vi "Enable Transient Operation.vi"(8 "error in (no error)":errorcluster, 10 "Enable Transient (T: Enable)":bool=TRUE, 11 "VISA resource name":refnum<visa-resource-name>) -> (0 "error out":errorcluster, 3 "VISA resource name out":refnum<visa-resource-name>)   [LabVIEW 2024, in "BK Precision 8500B Series.lvlib"]
doc: "Enable or disable the state of transient operation. Transient operation must be enabled first before sending a trigger to initiate the operation.\n\nRun this vi after configuring transient operation parameters using <b>Configure Transient Operation.vi</b>."
uses:
  BK Precision 8500B Series.lvlib
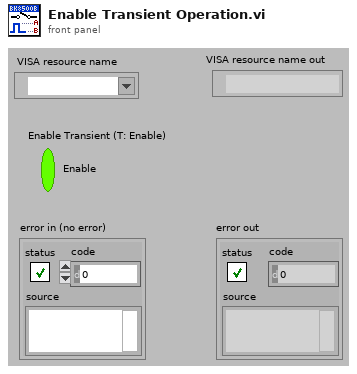
[diagram p1: front panel]
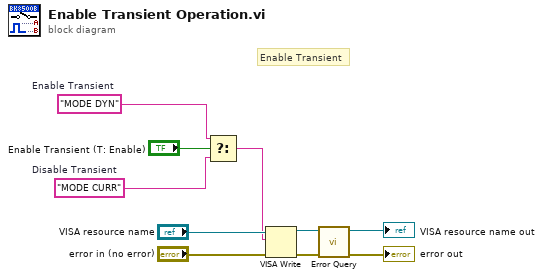
[diagram p0: block diagram]
diagram:
  w2 = "MODE DYN"  # Enable Transient
  w3 = "MODE CURR"  # Disable Transient
  # "Enable Transient"
  n1 = Select(t=w2, s="Enable Transient (T: Enable)", f=w3) -> (s? t:f=w1:string)
  n2 = VISA Write(VISA resource name="VISA resource name", write buffer=w1, error in (no error)="error in (no error)") -> (VISA resource name out=w7:refnum<visa-resource-name>, error out=w8:errorcluster)  [unwired: 1 out]
  n3 = call "Error Query.vi"("error in (no error)"=w8, "VISA resource name"=w7) -> ("error out"=→"error out":errorcluster, "VISA resource name out"=→"VISA resource name out":refnum<visa-resource-name>)  [unwired: 6 in, 2 out]
